vi "BGA244_set_gas_type.vi"(8 "error in":errorcluster, 9 "gas 2":string, 10 "gas 1":string, 11 "VISA in":refnum<visa-resource-name>="COM24") -> (0 "error out":errorcluster, 3 "VISA out":refnum<visa-resource-name>="COM24", 4 "status":bool=TRUE)   [LabVIEW 2019]
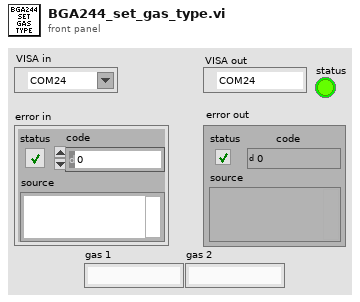
[diagram p1: front panel]
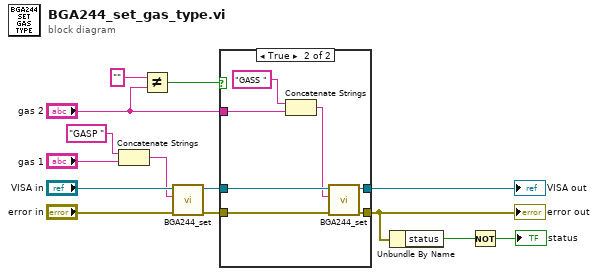
[diagram p0: block diagram]
diagram:
  n1 = Concatenate Strings("GASP " ("string"), "gas 1") -> (w4:string)
  n2 = Not Equal?(x="", y="gas 2") -> (x != y?=w1:bool)
  n3 = call "BGA244_set.vi"("error in"="error in", "string in"=w4, "VISA in"="VISA in") -> ("error out"=w10:errorcluster, "VISA out"=w12:refnum<visa-resource-name>)  [unwired: 7 in]
  n4 = case shown="True" w1 {
    tunnel: w12 -> [w16 w23]
    tunnel: [w16 w22] -> w11
    tunnel: w10 -> [w15 w21]
    tunnel: [w15 w20] -> w9
    tunnel: "gas 2" -> [_ w18]
    frame False {
    }
    frame True {
      n5 = Concatenate Strings("GASS " ("string"), w18) -> (w17:string)
      n6 = call "BGA244_set.vi"("error in"=w21, "string in"=w17, "VISA in"=w23) -> ("error out"=w20:errorcluster, "VISA out"=w22:refnum<visa-resource-name>)  [unwired: 7 in]
    }
  }
  "VISA out" <- w11
  "error out" <- w9
  n7 = Unbundle By Name(w9) -> ("status"=w8:bool)
  n8 = Not(x=w8) -> (.not. x?=→"status":bool)
